vi "Handle.vi"(8 "error in (no error)":errorcluster, 11 "Acquisition in":refnum<class "Acquisition.lvclass">) -> (0 "error out":errorcluster, 3 "Acquisition out":refnum<class "Acquisition.lvclass">)   [LabVIEW 2018, in "Acquisition.lvclass"]
uses:
  Acquisition.lvclass
  Acquisition.lvclass/Acquisition.ctl
  Device/Device.lvclass/Device.ctl
  Interface/Interface.lvclass/Interface.ctl
  Channel/Channel.lvclass
  C:/Users/devstaff/sparc4/s4gui/Versao ZeroMQ REQ-REP/SPARC4_GUI -20241111/Device/Device.lvclass
  Server/Server.lvclass
  Comm/Stream/Stream.lvclass
  Interface/Interface.lvclass
  Device/Device.lvclass
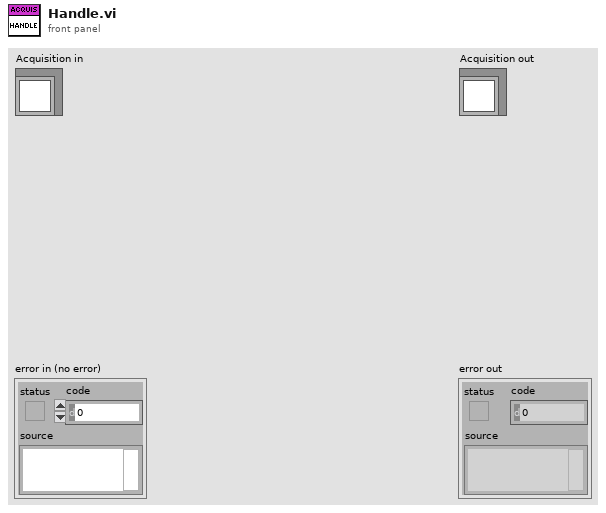
[diagram p1: front panel]
types:
  T1 = cluster{"ACQUISITION_MODE":u8, "TRIGGER_MODE":u8, "READ_MODE":u8, "PREAMP":u8, "READOUT_RATE":u8, "VERTICAL_SHIFT_SPEED":u8, "EM_MODE":u8, "EM_GAIN":u16, "SHUTTER_MODE":u8, "SHUTTER_TTL":u8, "SHUTTER_OPENING_TIME":u16, "SHUTTER_CLOSING_TIME":u16, "VBIN":u16, "HBIN":u16, "INITIAL_LINE":u16, "INITIAL_COLUMN":u16, "FINAL_LINE":u16, "FINAL_COLUMN":u16, "FRAME_TRANSFER":bool, "VERTICAL_CLOCK_VOLTAGE":u8, "AD_CHANNEL":u32}
  T2 = cluster{"ACQUISITION_MODE":bool, "TRIGGER_MODE":bool, "READ_MODE":bool, "PREAMP":bool, "READOUT_RATE":bool, "VERTICAL_SHIFT_SPEED":bool, "EM_MODE":bool, "EM_GAIN":bool, "SHUTTER_MODE":bool, "SHUTTER_TTL":bool, "SHUTTER_OPENING_TIME":bool, "SHUTTER_CLOSING_TIME":bool, "VBIN":bool, "HBIN":bool, "INITIAL_LINE":bool, "INITIAL_COLUMN":bool, "FINAL_LINE":bool, "FINAL_COLUMN":bool, "FRAME_TRANSFER":bool, "VERTICAL_CLOCK_VOLTAGE":bool, "AD_CHANNEL":bool}
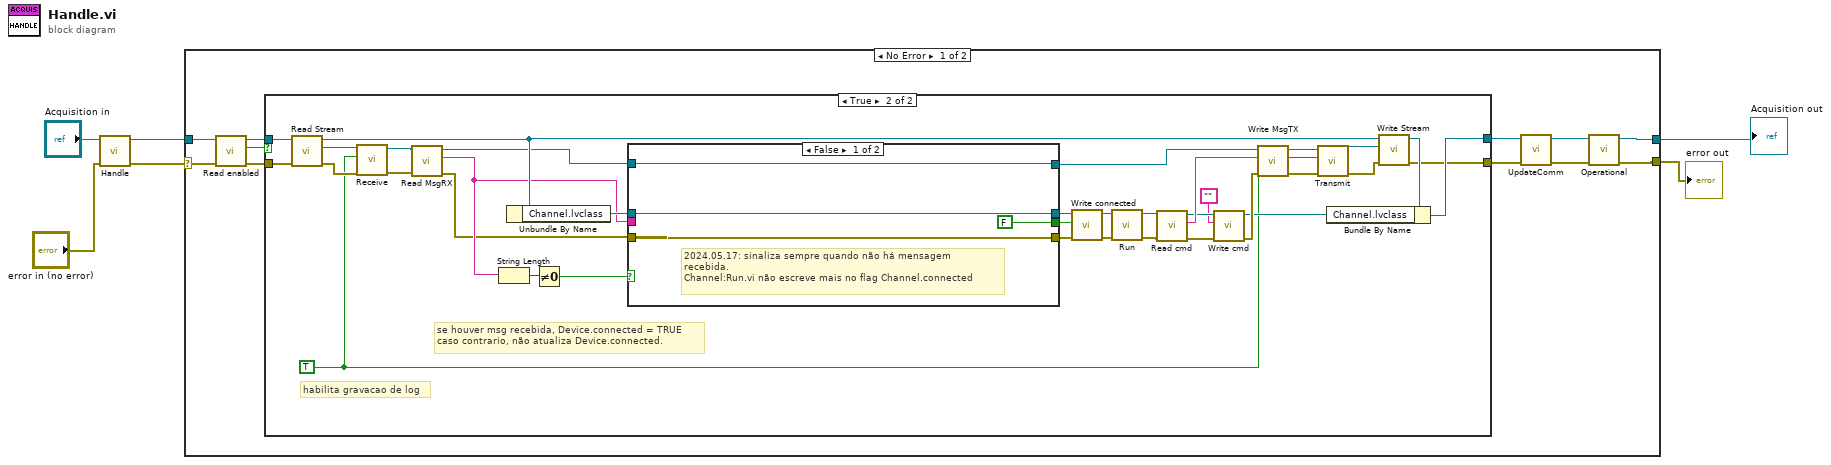
[diagram p0: block diagram]
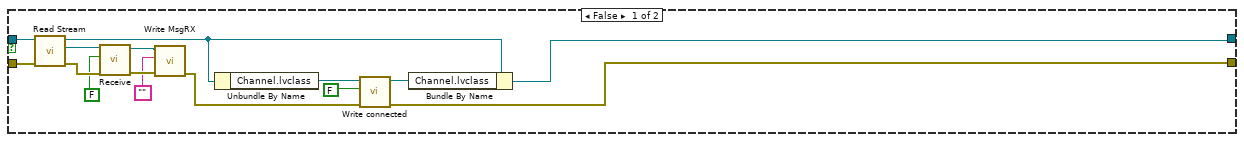
[diagram p2: hidden frame]
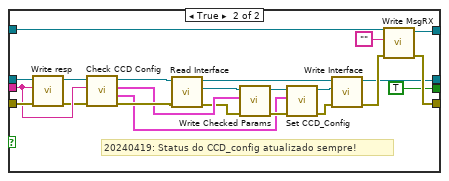
[diagram p3: hidden frame]
diagram:
  n1 = call-parent "Handle.vi"("error in (no error)"="error in (no error)", "Server in"="Acquisition in") -> ("error out"=w3:errorcluster, "Server out"=w4:refnum<class "Acquisition.lvclass">)  [unwired: 8 in]
  n2 = case shown="No Error" w3 {
    selector: w3 -> [w13 w96]
    tunnel: [w7 w96] -> w1
    tunnel: [w9 w95] -> w2
    tunnel: w4 -> [w15 w95]
    frame No Error {
      n3 = call-dynamic "Read enabled.vi"("error in (no error)"=w13, "Server in"=w15) -> ("error out"=w12:errorcluster, "enabled"=w11:bool, "Server out"=w14:refnum<class "Acquisition.lvclass">)  [unwired: 7 in]
      n4 = case shown="True" w11 {
        tunnel: w14 -> [w26 w67]
        tunnel: w12 -> [w25 w64]
        tunnel: [w20 w44] -> w17
        tunnel: [w18 w43] -> w16
        frame False {
          n5 = call-dynamic "Read Stream.vi"("error in (no error)"=w25, "Server in"=w26) -> ("error out"=w31:errorcluster, "Stream.lvclass"=w32:refnum<class "Stream.lvclass">, "Server out"=w21:refnum<class "Acquisition.lvclass">)  [unwired: 7 in]
          n6 = call-dynamic "Receive.vi"("error in (no error)"=w31, "log?"=FALSE, "Stream in"=w32) -> ("error out"=w30:errorcluster, "Stream out"=w29:refnum<class "Stream.lvclass">)  [unwired: 7 in]
          n7 = call-dynamic "Write MsgRX.vi"("error in (no error)"=w30, "MsgRX"="", "Comm in"=w29) -> ("error out"=w19:errorcluster)  [unwired: 7 in, 1 out]
          n8 = Unbundle By Name(w21) -> ("Channel.lvclass"=w24:refnum<class "Channel.lvclass">)
          n9 = call "Write connected.vi"("error in (no error)"=w19, "connected"=FALSE, "Device in"=w24) -> ("error out"=w18:errorcluster, "Device out"=w22:refnum<class "Channel.lvclass">)  [unwired: 7 in]
          n10 = Bundle By Name(cluster=w21, "Channel.lvclass"=w22) -> (w20:refnum<class "Acquisition.lvclass">)
        }
        frame True {
          w42 = TRUE ("log?")
          # "habilita gravacao de log"
          # "se houver msg recebida, Device.connected = TRUE\ncaso contrario, não atualiza Device.connected."
          n11 = call-dynamic "Read Stream.vi"("error in (no error)"=w64, "Server in"=w67) -> ("error out"=w65:errorcluster, "Stream.lvclass"=w66:refnum<class "Stream.lvclass">, "Server out"=w58:refnum<class "Acquisition.lvclass">)  [unwired: 7 in]
          n12 = call-dynamic "Receive.vi"("error in (no error)"=w65, "log?"=w42, "Stream in"=w66) -> ("error out"=w63:errorcluster, "Stream out"=w62:refnum<class "Stream.lvclass">)  [unwired: 7 in]
          n13 = call-dynamic "Read MsgRX.vi"("error in (no error)"=w63, "Comm in"=w62) -> ("error out"=w47:errorcluster, "MsgRX"=w48:string, "Comm out"=w41:refnum<class "Stream.lvclass">)  [unwired: 7 in]
          n14 = String Length(string=w48) -> (length=w52:i32)
          n15 = Unbundle By Name(w58) -> ("Channel.lvclass"=w49:refnum<class "Channel.lvclass">)
          n16 = Not Equal To 0?(x=w52) -> (x != 0?=w46:bool)
          n17 = case shown="False" w46 {
            tunnel: w47 -> [w70 w86]
            tunnel: w49 -> [w71 w94]
            tunnel: [w71 w73] -> w37
            tunnel: [w70 w85] -> w35
            tunnel: w48 -> [_ w81]
            tunnel: w41 -> [w69 w93]
            tunnel: [w69 w92] -> w40
            tunnel: [FALSE TRUE] -> w33
            frame False {
              # "2024.05.17: sinaliza sempre quando não há mensagem \nrecebida. \nChannel:Run.vi não escreve mais no flag Channel.connected"
            }
            frame True {
              # "20240419: Status do CCD_config atualizado sempre!"
              n18 = call-dynamic "Write resp.vi"("error in (no error)"=w86, "resp"=w81, "Device in"=w94) -> ("error out"=w80:errorcluster, "Device out"=w82:refnum<class "Channel.lvclass">)  [unwired: 7 in]
              n19 = call-dynamic "Check CCD Config.vi"("error in (no error)"=w80, "Status"=w81, "Channel in"=w82) -> ("error out"=w78:errorcluster, "cluster RX"=w75:T1, "Cluster COMPARE"=w77:T2, "Channel out"=w79:refnum<class "Channel.lvclass">)  [unwired: 5 in]
              n20 = call-dynamic "Read Interface.vi"("error in (no error)"=w78, "Channel in"=w79) -> ("error out"=w76:errorcluster, "Interface.lvclass"=w83:refnum<class "Interface.lvclass">, "Channel out"=w90:refnum<class "Channel.lvclass">)  [unwired: 7 in]
              n21 = call "Write Checked Params.vi"("error in (no error)"=w76, "Checked Params"=w77, "Interface in"=w83) -> ("error out"=w88:errorcluster, "Interface out"=w89:refnum<class "Interface.lvclass">)  [unwired: 7 in]
              n22 = call-dynamic "Set CCD_Config.vi"("error in (no error)"=w88, "input cluster"=w75, "Interface in"=w89) -> ("error out"=w87:errorcluster, "Interface out"=w84:refnum<class "Interface.lvclass">)  [unwired: 7 in]
              n23 = call-dynamic "Write Interface.vi"("error in (no error)"=w87, "Interface.lvclass"=w84, "Channel in"=w90) -> ("error out"=w74:errorcluster, "Channel out"=w73:refnum<class "Channel.lvclass">)  [unwired: 7 in]
              n24 = call-dynamic "Write MsgRX.vi"("error in (no error)"=w74, "MsgRX"="", "Comm in"=w93) -> ("error out"=w85:errorcluster, "Comm out"=w92:refnum<class "Stream.lvclass">)  [unwired: 7 in]
            }
          }
          n25 = call "Write connected.vi"("error in (no error)"=w35, "connected"=w33, "Device in"=w37) -> ("error out"=w34:errorcluster, "Device out"=w36:refnum<class "Channel.lvclass">)  [unwired: 7 in]
          n26 = call-dynamic "Run.vi"("error in (no error)"=w34, "Channel in"=w36) -> ("error out"=w38:errorcluster, "Channel out"=w39:refnum<class "Channel.lvclass">)  [unwired: 8 in]
          n27 = call-dynamic "Read cmd.vi"("error in (no error)"=w38, "Device in"=w39) -> ("error out"=w54:errorcluster, "cmd"=w61:string, "Device out"=w55:refnum<class "Channel.lvclass">)  [unwired: 7 in]
          n28 = call-dynamic "Write cmd.vi"("error in (no error)"=w54, "cmd"="", "Device in"=w55) -> ("error out"=w51:errorcluster, "Device out"=w50:refnum<class "Channel.lvclass">)  [unwired: 7 in]
          n29 = call-dynamic "Write MsgTX.vi"("error in (no error)"=w51, "MsgTX"=w61, "Comm in"=w40) -> ("error out"=w59:errorcluster, "Comm out"=w60:refnum<class "Stream.lvclass">)  [unwired: 7 in]
          n30 = call-dynamic "Transmit.vi"("error in (no error)"=w59, "log?"=w42, "Stream in"=w60) -> ("error out"=w56:errorcluster, "Stream out"=w57:refnum<class "Stream.lvclass">)  [unwired: 7 in]
          n31 = call-dynamic "Write Stream.vi"("error in (no error)"=w56, "Stream.lvclass"=w57, "Server in"=w58) -> ("error out"=w43:errorcluster, "Server out"=w45:refnum<class "Acquisition.lvclass">)  [unwired: 7 in]
          n32 = Bundle By Name(cluster=w45, "Channel.lvclass"=w50) -> (w44:refnum<class "Acquisition.lvclass">)
        }
      }
      n33 = call-dynamic "UpdateComm.vi"("error in (no error)"=w16, "Acquisition in"=w17) -> ("error out"=w8:errorcluster, "Acquisition out"=w10:refnum<class "Acquisition.lvclass">)  [unwired: 8 in]
      n34 = call-dynamic "Operational.vi"("error in (no error)"=w8, "Acquisition in"=w10) -> ("error out"=w7:errorcluster, "Acquisition out"=w9:refnum<class "Acquisition.lvclass">)  [unwired: 8 in]
    }
    frame Error {
    }
  }
  "error out" <- w1
  "Acquisition out" <- w2
